vi "Get Fields.vi"(11 "Info Section in":refnum<class "Info Section.lvclass">) -> (2 "Fields Cluster":variant, 3 "Info Section out":refnum<class "Info Section.lvclass">)   [LabVIEW 2024, in "Electronic Datasheet.lvlib" / "Info Section.lvclass"]
uses:
  Info Section.lvclass
  Info Section.lvclass/Info Section.ctl
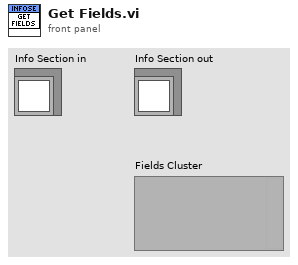
[diagram p1: front panel]
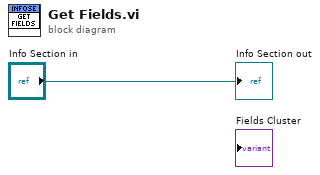
[diagram p0: block diagram]
diagram:
  "Info Section out" <- "Info Section in"
